vi "Process Platform Via.vi"(8 "error in (no error)":errorcluster, 10 "Raw VIA":string, 11 "RP2040Platform in":refnum<class "RP2040Platform.lvclass">) -> (0 "error out":errorcluster, 2 "VIA":string, 3 "RP2040Platform out":refnum<class "RP2040Platform.lvclass">)   [LabVIEW 2020, in "RP2040.lvlib" / "RP2040Platform.lvclass"]
uses:
  RP2040Platform.lvclass
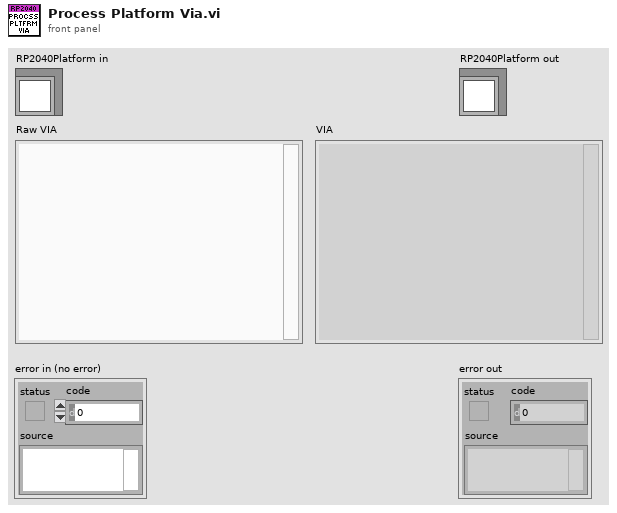
[diagram p1: front panel]
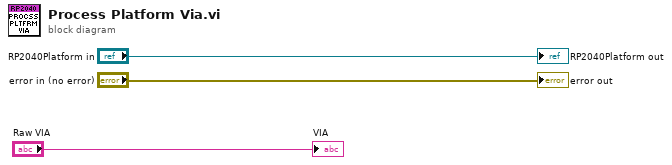
[diagram p0: block diagram]
diagram:
  "error out" <- "error in (no error)"
  "RP2040Platform out" <- "RP2040Platform in"
  "VIA" <- "Raw VIA"
